vi "Add Edit Chan Group.vi"(8 "error in (no error)":errorcluster, 10 "Add (F) / Edit (T)":bool, 11 "Cfg Grandmaster in":refnum<class "Cfg Grandmaster.lvclass">) -> (0 "error out":errorcluster, 3 "Cfg Grandmaster out":refnum<class "Cfg Grandmaster.lvclass">)   [LabVIEW 2018, in "Configuration Grandmaster.lvlib" / "Cfg Grandmaster.lvclass"]
uses:
  Cfg Grandmaster.lvclass
  Cfg Grandmaster.lvclass/Cfg Grandmaster.ctl
  Common/Controls/Selected Group.ctl
  Common/Controls/TE_Designator.ctl
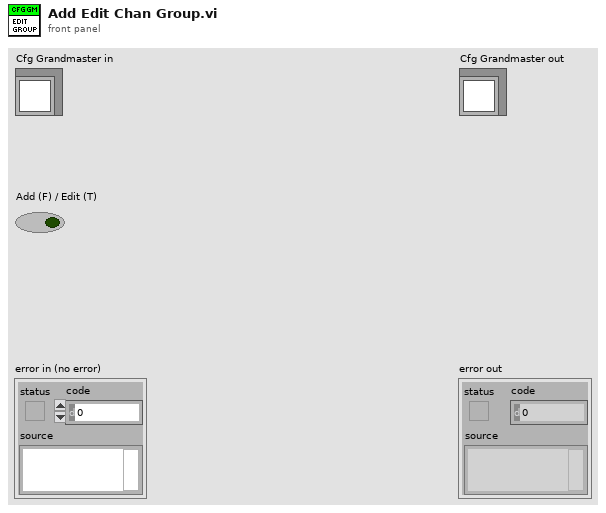
[diagram p1: front panel]
types:
  T1 = typedef "Selected Group.ctl" = cluster{"ChanGroup":i32, "Rate Class":T2}
  T2 = typedef "TE_Designator.ctl" = enum16{"High Speed", "Low Speed"}
  T3 = typedef "ge_Cfg wChassis.ctl" = cluster{"Chassis BOM":refnum<class "Chassis BOM.lvclass">, "Chassis Cfg":refnum<class "ChassisCfg.lvclass">, "Chassis Tasks":refnum<class "Chassis Tasks.lvclass">, "HW Error":bool, "Unsvd Chgs?":bool}
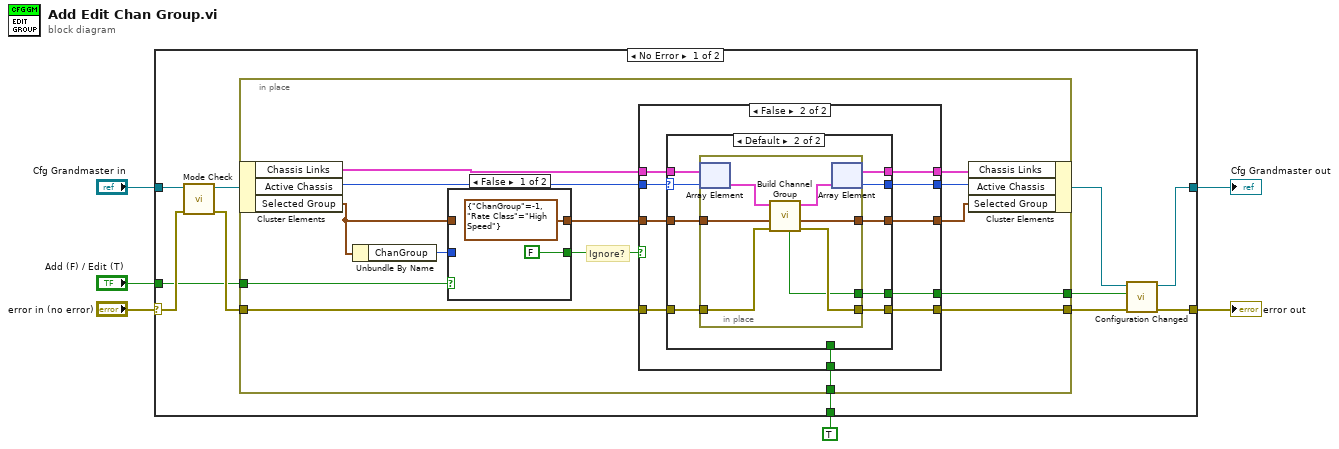
[diagram p0: block diagram]
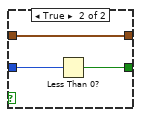
[diagram p2: hidden frame]
diagram:
  n1 = case shown="No Error" "error in (no error)" {
    selector: "error in (no error)" -> [w13 w74]
    tunnel: [w10 w74] -> w5
    tunnel: [w9 w73] -> w3
    tunnel: "Cfg Grandmaster in" -> [w16 w73]
    tunnel: TRUE ("Canceled?") -> [w17 _]
    tunnel: "Add (F) / Edit (T)" -> [w7 _]
    frame No Error {
      n2 = call "Mode Check.vi"("error in (no error)"=w13, "Cfg Grandmaster in"=w16) -> ("error out"=w14:errorcluster, "Cfg Grandmaster out"=w15:refnum<class "Cfg Grandmaster.lvclass">)  [unwired: 8 in]
      n3 = in-place {
        in-place-border: w14 -> [w27]
        in-place-border: [w26] -> w11
        in-place-border: w17 -> [w25]
        in-place-border: [w23] -> w8
        in-place-border: w7 -> [w22]
        # "Ignore?"
        n4 = in-place-cluster #1(w15) -> ("Chassis Links"=w31:T3[], "Active Chassis"=w30:i32, "Selected Group"=w19:T1)
        n5 = Unbundle By Name(w19) -> ("ChanGroup"=w21:i32)
        n6 = case shown="False" w22 {
          tunnel: w21 -> [_ w35]
          tunnel: [T1 {"ChanGroup"=-1, "Rate Class"=enum."High Speed"} ("Selected Group") w36] -> w20
          tunnel: w19 -> [_ w36]
          tunnel: [FALSE w34] -> w18
          frame False {
          }
          frame True {
            n7 = Less Than 0?(x=w35) -> (x < 0?=w34:bool)
          }
        }
        n8 = case shown="False" w18 {
          tunnel: w27 -> [w40 w51]
          tunnel: [w40 w50] -> w26
          tunnel: [w41 w49] -> w24
          tunnel: w20 -> [w41 w48]
          tunnel: w31 -> [w39 w47]
          tunnel: [w39 w46] -> w29
          tunnel: w30 -> [w37 w44]
          tunnel: [w38 w45] -> w23
          tunnel: w25 -> [w38 w43]
          tunnel: [w37 w42] -> w28
          frame True {
          }
          frame False {
            n9 = case shown="Default" w44 {
              selector: w44 -> [w52 w58]
              tunnel: w51 -> [w54 w65]
              tunnel: [w54 w64] -> w50
              tunnel: [w55 w63] -> w49
              tunnel: w48 -> [w55 w62]
              tunnel: w47 -> [w56 w61]
              tunnel: [w56 w60] -> w46
              tunnel: [w53 w59] -> w45
              tunnel: w43 -> [w53 _]
              tunnel: [w52 w57] -> w42
              frame -1 {
              }
              frame Default {
                n10 = in-place {
                  in-place-border: w65 -> [w72]
                  in-place-border: [w71] -> w64
                  in-place-border: [w70] -> w63
                  in-place-border: w62 -> [w69]
                  in-place-border: [w68] -> w59
                  n11 = in-place-array #2(w61, w58) -> (w67:T3)
                  n12 = call "Build Channel Group.vi"("error in"=w72, "Selected Group"=w69, "Config Grandmaster"=w67) -> ("error out"=w71:errorcluster, "Selected Group"=w70:T1, "Config Grandmaster"=w66:T3, "Canceled?"=w68:bool)  [unwired: 5 in]
                  n13 = in-place-array #2(w66) -> (w60:T3[], w57:i32)
                }
              }
            }
          }
        }
        n14 = in-place-cluster #1("Chassis Links"=w29, "Active Chassis"=w28, "Selected Group"=w24) -> (w12:refnum<class "Cfg Grandmaster.lvclass">)
      }
      n15 = call "Configuration Changed.vi"("error in (no error)"=w11, "Canceled? (F)"=w8, "Cfg Grandmaster in"=w12) -> ("error out"=w10:errorcluster, "Cfg Grandmaster out"=w9:refnum<class "Cfg Grandmaster.lvclass">)  [unwired: 7 in]
    }
    frame Error {
    }
  }
  "error out" <- w5
  "Cfg Grandmaster out" <- w3
